vi "Variant Icon Name.vi"(8 "Error In":errorcluster, 11 "Value":variant) -> (0 "Error Out":errorcluster, 3 "String":string)   [LabVIEW 2018, in "Scripts.lvlib"]
uses:
  Scripts.lvlib
  <vilib>/Utility/Data Type/NI_Data Type.lvlib
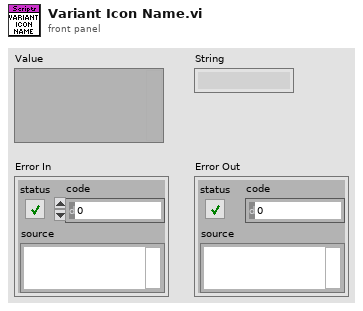
[diagram p1: front panel]
types:
  T1 = typedef "NI_Data Type.lvlib/Data Type.ctl" = enum8{"Invalid Type", "Void", "I8", "I16", "I32", "I64", "U8", "U16", "U32", "U64", "Single Float", "Double Float", "Extended Float", "Single Complex", "Double Complex", "Extended Complex", "Enum U8", "Enum U16", "Enum U32", "Enum U64", "Single Float With Unit", "Double Float With Unit", "Extended Float With Unit", "Single Complex with Unit", "Double Complex with Unit", "Extended Complex with Unit", "Boolean", "String", "Path", "Picture", "Tag", "Array", "Cluster", "Variant", "LV Variant", "Waveform", "Timestamp", "Digital Waveform", "Digital Data", "ExpressData", "Refnum", "External Data", "VI", "Poly VI", "LabVIEW Class Instance", "Fixed Point"}
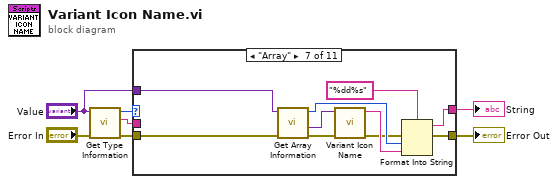
[diagram p0: block diagram]
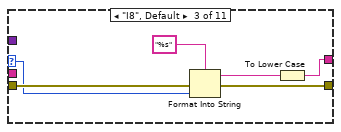
[diagram p4: hidden frame]
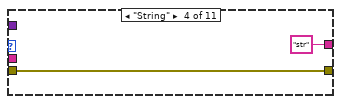
[diagram p5: hidden frame]
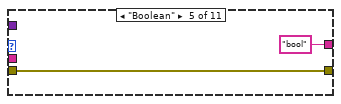
[diagram p6: hidden frame]
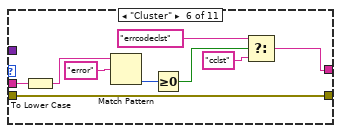
[diagram p7: hidden frame]
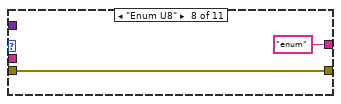
[diagram p8: hidden frame]
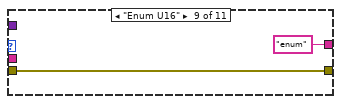
[diagram p9: hidden frame]
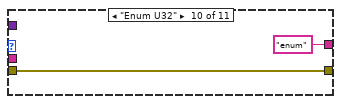
[diagram p10: hidden frame]
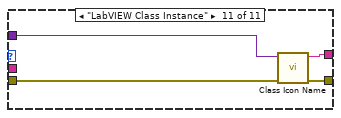
[diagram p11: hidden frame]
diagram:
  n1 = call <vilib>:"Get Type Information.vi"("error in (no error)"="Error In", "Variant"="Value") -> ("error out"=w4:errorcluster, "Name"=w6:string, "Type"=w2:T1)  [unwired: 5 in, 2 out]
  n2 = case shown="\"Array\"" w2 {
    selector: w2 -> [_ _ w12 _ _ _ _ _ _ _ _]
    tunnel: [_ _ w10 "str" "bool" w21 w33 "enum" ("f") "enum" ("f") "enum" ("f") w45] -> w3
    tunnel: w4 -> [w8 w9 w15 w17 w19 w28 w37 w40 w42 w44 w47]
    tunnel: [w8 w9 w14 w17 w19 w28 w34 w40 w42 w44 w46] -> w5
    tunnel: w6 -> [_ _ _ _ _ w27 _ _ _ _ _]
    tunnel: "Value" -> [_ _ _ _ _ _ w38 _ _ _ w48]
    frame "Invalid Type" {
    }
    frame "Void" {
    }
    frame "I8", Default {
      n3 = Format Into String(format string="%s", error in=w15, w12) -> (resulting string=w11:string, error out=w14:errorcluster)  [unwired: 1 in]
      n4 = To Lower Case(string=w11) -> (all lower case string=w10:string)
    }
    frame "String" {
    }
    frame "Boolean" {
    }
    frame "Cluster" {
      n5 = To Lower Case(string=w27) -> (all lower case string=w26:string)
      n6 = Match Pattern(string=w26, regular expression="error") -> (offset past match=w24:i32)  [unwired: 1 in, 3 out]
      n7 = Greater Or Equal To 0?(x=w24) -> (x >= 0?=w23:bool)
      n8 = Select(t="errcodeclst", s=w23, f="cclst") -> (s? t:f=w21:string)
    }
    frame "Array" {
      n9 = call <vilib>:"Get Array Information.vi"("error in (no error)"=w37, "Variant"=w38) -> ("error out"=w31:errorcluster, "Array Element Data Type"=w32:variant, "Number of Dimensions"=w35:i32)  [unwired: 6 in, 1 out]
      n10 = call "Variant Icon Name.vi"("Error In"=w31, "Value"=w32) -> ("Error Out"=w29:errorcluster, "String"=w30:string)  [unwired: 8 in]
      n11 = Format Into String(format string="%dd%s", error in=w29, w35, w30) -> (resulting string=w33:string, error out=w34:errorcluster)  [unwired: 1 in]
    }
    frame "Enum U8" {
    }
    frame "Enum U16" {
    }
    frame "Enum U32" {
    }
    frame "LabVIEW Class Instance" {
      n12 = call "Class Icon Name.vi"("Error In"=w47, "Value"=w48) -> ("Error Out"=w46:errorcluster, "String"=w45:string)  [unwired: 8 in]
    }
  }
  "Error Out" <- w5
  "String" <- w3
